vi "USRP Dummy (FPGA).vi"() -> ()   [LabVIEW 2016]
uses:
  <instrlib>/_niInstr/Register Bus/v1/FPGA/Public/Read Cmd Data.ctl
  <vilib>/Platform/TimedLoop/XDataNode/timing_clust.ctl
  <vilib>/Platform/TimedLoop/XDataNode/nitl_modes.ctl
  <vilib>/Platform/TimedLoop/XDataNode/wakeup.ctl
  <vilib>/rvi/Emulation/niFpgaSctlEmulationGetInTimedLoop.vi
  <vilib>/rvi/Emulation/niFpgaEmulationReportErrorSimple.vi
  <vilib>/rvi/Emulation/niFpgaGetClockAttributes.vi
  <vilib>/rvi/Emulation/niFpgaCriticalErrorInLSC.vi
  <vilib>/rvi/eio/common/nirviEmuTemplateMethod_errors.vi
  <vilib>/rvi/interface/RandomDataEmulation/niFpgaRandomDataHandleErrors.vi
  <vilib>/Platform/TimedLoop/XDataNode/XDataNode.xnode
  <vilib>/eio/EIONode/EIONode.xnode
  <vilib>/rvi/DataTransferAndStorage/Container/XNode/niFpgaContainer.xnode
  <vilib>/rvi/interface/RandomDataEmulation/nirviRandomDataFpgaReadWriteTemplate.vi
  <vilib>/Platform/TimedLoop/XDataNode/XDNodeRunTimeDep.lvlib
  <instrlib>/_niInstr/Register Bus/v1/FPGA/niInstr Register Bus v1 FPGA.lvlib
  <instrlib>/niUsrpRio/Config/v1/FPGA/niUsrpRio Config v1 FPGA.lvlib
  <instrlib>/_niInstr/Basic Elements/v1/FPGA/niInstr Basic Elements v1 FPGA.lvlib
panel:
  out "Min Space Available":u32
  out "Space Available":u32
  in  "Simulated Data Type":enum16{"Sequential", "Pseudo Random"}(ring)
  out "FPGA FIFO Depth":u32
  in  "Reset FPGA Transfer Count?":bool
  out "Send Status?":bool
  out "Samples Left to Write":u64
  in  "Number of Samples":u64
  in  "reg.host read.go rcvd 0":bool
  out "reg.notify host.go 0":bool
  in  "reg.notify host.go rcvd 0":bool
  out "reg.host read.data 0":T1
  in  "reg.reset 0":bool
  in  "RF 0/Rx/Enable":bool
  in  "RF 0/Tx/Enable":bool
  in  "RF 1/Rx/Enable":bool
  in  "RF 1/Tx/Enable":bool
  out "FPGA Transfer Count":u64
  in  "Send Data?":bool
  in  "Reset Total Timeouts?":bool
  out "Total Timeouts":u64
  out "Sticky Timeout?":bool
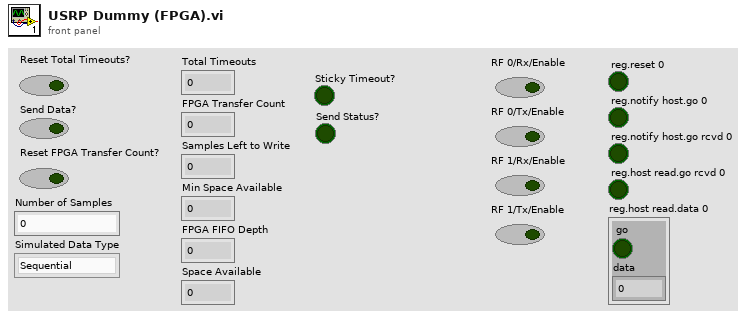
[diagram p1: front panel]
types:
  T1 = typedef "niInstr Register Bus v1 FPGA.lvlib/Read Cmd Data.ctl" = cluster{"go":bool, "data":u32}
  T2 = typedef "XDNodeRunTimeDep.lvlib/timing_clust.ctl" = cluster{"Expected End [f-1]":u64, "Actual End [f-1]":u64, "Finished Late? [f-1]":bool, "Expected End [i-1]":u64, "Actual End [i-1]":u64, "Finished Late? [i-1]":bool, "Expected Start [i]":u64, "Actual Start [i]":u64, "Expected Start [f]":u64, "Actual Start [f]":u64, "Source Name":string, "Structure Name":string, "Period":i64, "Deadline":i64, "Offset":i64, "Start":i64, "Priority":i32, "Timeout":i32, "Mode":T3, "Wakeup Reason":T4, "Error":errorcluster, "Source Type":string, "Secondary Source Type":string, "Global End Time":u64, "Global Start Time":u64, "Frame Duration":u64, "Iteration Duration":u64, "Assigned CPU":i32, "I/O Scan Engine Mode":u32}
  T3 = typedef "XDNodeRunTimeDep.lvlib/nitl_modes.ctl" = enum32{"No Change", "Process missed periods, maintain original phase", "Discard missed periods, maintain original phase", "Process missed periods, ignore original phase", "Discard missed periods, ignore original phase"}
  T4 = typedef "XDNodeRunTimeDep.lvlib/wakeup.ctl" = enum32{"Normal", "Aborted", "Asynchronous wakeup", "Timing source error", "Timed loop error", "Timeout"}
  T5 = cluster{"DAC FIFO Reset":refnum<k21>, "RF 0 Rx Swap IQ":refnum<k21>, "RF 0 Rx Negate I":refnum<k21>, "RF 0 Rx Negate Q":refnum<k21>, "RF 0 Rx Data Valid":refnum<k21>, "RF 0 Rx Data Ever Invalid":refnum<k21>, "clear RF 0 Rx Data Ever Invalid":refnum<k21>, "RF 0 Tx Swap IQ":refnum<k21>, "RF 0 Tx Negate I":refnum<k21>, "RF 0 Tx Negate Q":refnum<k21>, "RF 1 Rx Swap IQ":refnum<k21>, "RF 1 Rx Negate I":refnum<k21>, "RF 1 Rx Negate Q":refnum<k21>, "RF 1 Rx Data Valid":refnum<k21>, "RF 1 Rx Data Ever Invalid":refnum<k21>, "clear RF 1 Rx Data Ever Invalid":refnum<k21>, "RF 1 Tx Swap IQ":refnum<k21>, "RF 1 Tx Negate I":refnum<k21>, "RF 1 Tx Negate Q":refnum<k21>}
  T6 = typedef "niUsrpRio Synchronization v1 FPGA.lvlib/Resources.ctl" = cluster{"master":refnum<k21>, "meas.enable":refnum<k21>, "meas.ready":refnum<k21>, "meas.reset":refnum<k21>, "meas.arm":refnum<k21>, "meas.valid":refnum<k21>, "meas.value":refnum<k21>, "meas.oversample factor":refnum<k21>, "cptr":refnum<k21>, "cptr.adjust":refnum<k21>, "cptr.period":refnum<k21>}
  T7 = typedef "niUsrpRio Time v1 FPGA.lvlib/Time Resources.ctl" = cluster{"reset":refnum<k21>, "time":refnum<k21>, "time.previous cptr":refnum<k21>, "new time":refnum<k21>, "new time.when":refnum<k21>, "new time.set":refnum<k21>, "which edge of ref":refnum<k21>, "pps source":refnum<k21>, "internal pps period":refnum<k21>}
  T8 = typedef "niUsrpRio Time v1 FPGA.lvlib/Future Event Resources.ctl" = cluster{"reset":refnum<k21>, "future event.time":refnum<k21>, "future event.ready":refnum<k21>, "future event.set":refnum<k21>, "future event.clear":refnum<k21>, "future event.set in past":refnum<k21>}
  T9 = cluster{"time.resources":T7, "future event.resources":T8, "future event.resources":T8, "future event.resources":T8}
  T10 = typedef "niInstr Register Bus v1 FPGA.lvlib/Register Instruction.ctl" = cluster{"subsystem":u8, "address":u16, "data":u32, "valid":bool, "read":bool}
  T11 = typedef "niInstr Register Bus v1 FPGA.lvlib/Read Completion.ctl" = cluster{"data":u32, "valid":bool}
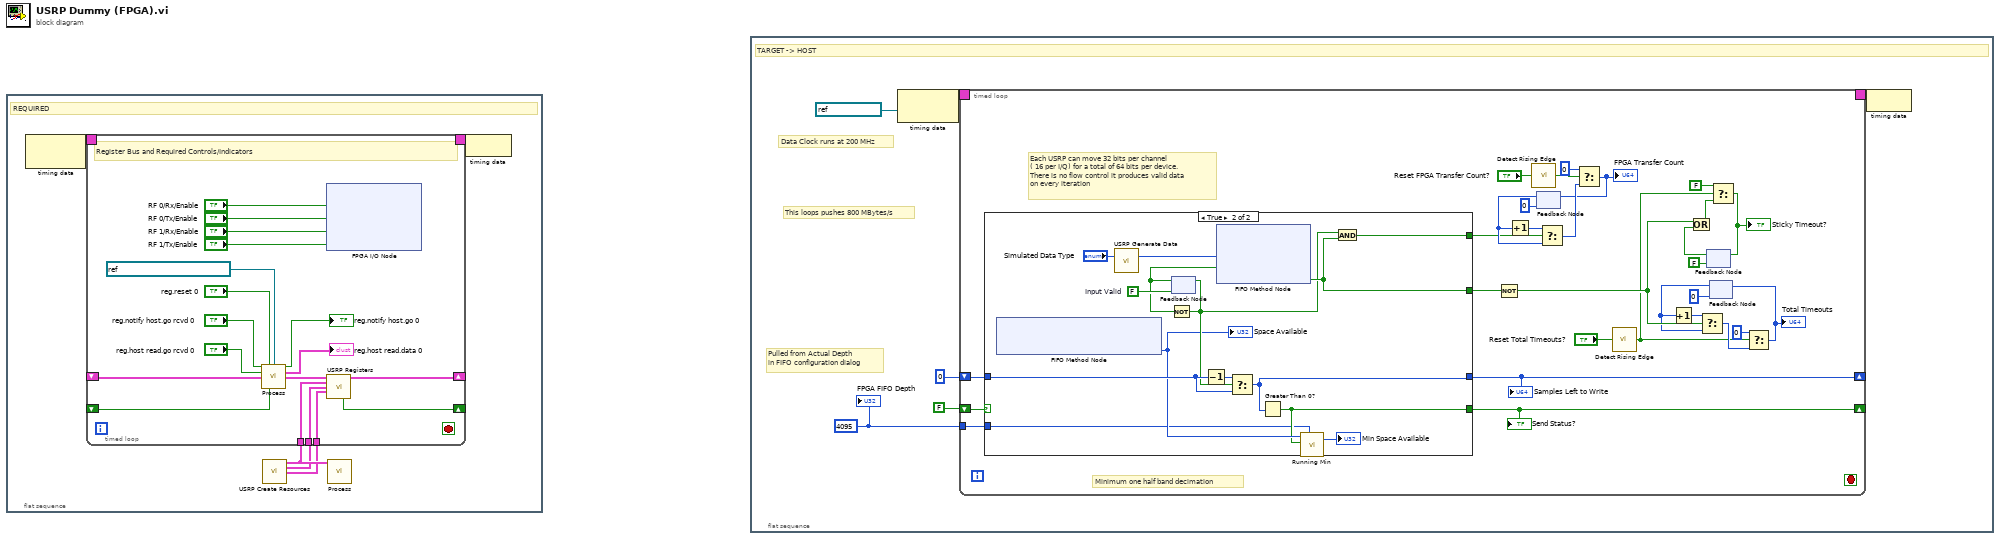
[diagram p0: block diagram]
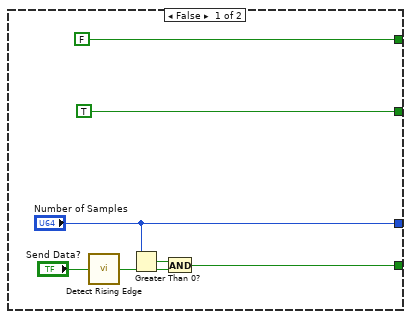
[diagram p2: hidden frame]
diagram:
  n1 = flat-sequence {
    frame #0 {
      # "REQUIRED"
      n2 = node-c288() -> (w5:T2)  [unwired: 1 in]
      n3 = call "USRP Create Resources.vi"() -> ("config.resources"=w3:T5, "sync.resources"=w2:T6, "time.resources"=w1:T9)  [unwired: 13 in]
      n4 = timed-loop "Register Bus and Required Controls/Indicators" {
        timing: w5 -> [_]
        timing-out: [_] -> w4
        shift-right: [w20] -> _
        shift-left: _ -> [w19]
        shift-right: [w14] -> _
        shift-left: _ -> [w18]
        tunnel: w3 -> [w12]
        tunnel: w2 -> [w11]
        tunnel: w1 -> [w10]
        stop <- _ stop-if-true
        # "Register Bus and Required Controls/Indicators"
        n5 = call <instrlib>:"Process.vi"("reg.notify host.go rcvd"="reg.notify host.go rcvd 0", "reg.reset"="reg.reset 0", "reg.host instruction fifo"=refnum<k21> "reg.host instruction fifo 0", "reg.host read.go rcvd"="reg.host read.go rcvd 0", "read completion"=w19, "ready for output"=w18) -> ("reg.notify host.go"=→"reg.notify host.go 0":bool, "reg.host read.data"=→"reg.host read.data 0":T1, "register instruction"=w13:T10)  [unwired: 7 in]
        n6 = xnode ("FPGA I/O Node")("RF 0/Rx/Enable"="RF 0/Rx/Enable", "RF 0/Tx/Enable"="RF 0/Tx/Enable", "RF 1/Rx/Enable"="RF 1/Rx/Enable", "RF 1/Tx/Enable"="RF 1/Tx/Enable") -> ()  [unwired: 4 in, 4 out]
        n7 = call "USRP Registers.vi"("register instruction"=w13, "config.resources"=w12, "sync.resources"=w11, "time.resources"=w10) -> ("read completion out"=w20:T11, "ready for input"=w14:bool)  [unwired: 10 in]
      }
      n8 = call <instrlib>:"Process.vi"("resources"=w3) -> ()  [unwired: 15 in]
      n9 = node-c288(w4) -> ()
    }
  }
  n10 = flat-sequence {
    frame #0 {
      w28 = u32 4095 ("FPGA FIFO Depth")
      # "Pulled from Actual Depth\nin FIFO configuration dialog"
      # "This loops pushes 800 MBytes/s"
      # "Data Clock runs at 200 MHz"
      # "TARGET -> HOST"
      n11 = node-c288(refnum<k21> "Data Clock" ("Source Name")) -> (w33:T2)
      n12 = timed-loop {
        timing: w33 -> [_]
        timing-out: [_] -> w32
        shift-right: [w50] -> _
        shift-left: FALSE ("send data?") -> [w49]
        shift-right: [w47] -> _
        shift-left: u64 0 ("samples to write") -> [w48]
        tunnel: w28 -> [w38]
        stop <- _ stop-if-true
        # "Each USRP can move 32 bits per channel\n( 16 per I/Q) for a total of 64 bits per device.\nThere is no flow control it produces valid data\non every iteration"
        # "Minimum one half band decimation"
        n13 = case shown="True" w49 {
          tunnel: [FALSE ("Timed Out?") w75] -> w53
          tunnel: [TRUE ("Timed Out?") w83] -> w52
          tunnel: [w65 w72] -> w50
          tunnel: w48 -> [_ w78]
          tunnel: ["Number of Samples" w79] -> w47
          tunnel: w38 -> [_ w71]
          frame False {
            n14 = call <instrlib>:"Detect Rising Edge.vi"("signal"="Send Data?") -> ("edge detected"=w66:bool)  [unwired: 14 in]
            n15 = Greater Than 0?(x="Number of Samples") -> (x > 0?=w64:bool)
            n16 = And(x=w64, y=w66) -> (x .and. y?=w65:bool)
          }
          frame True {
            w82 = FALSE  # Input Valid
            n17 = xnode ("FIFO Method Node")() -> ("Number of Elements to Write"=w73:u32)  [unwired: 1 in, 1 out]
            "Space Available" <- w73
            n18 = call "USRP Generate Data.vi"("Enum"="Simulated Data Type") -> ("Data"=w77:u64)  [unwired: 14 in]
            n19 = feedback #1(w82) -> (w81:bool)
            n20 = Not(x=w81) -> (.not. x?=w74:bool)
            n21 = feedback-in #1(w74) -> ()
            n22 = Decrement(x=w78) -> (x-1=w80:u64)
            n23 = xnode ("FIFO Method Node")("Element"=w77, "Input Valid"=w81) -> ("Ready for Input"=w83:bool)  [unwired: 1 in, 1 out]
            n24 = Select(t=w80, s=w74, f=w78) -> (s? t:f=w79:u64)
            n25 = Greater Than 0?(x=w79) -> (x > 0?=w72:bool)
            n26 = call "Running Min.vi"("Starting Min"=w71, "Reset"=w72, "Next Value"=w73) -> ("Running Min"=→"Min Space Available":u32)  [unwired: 4 in]
            n27 = And(x=w74, y=w83) -> (x .and. y?=w75:bool)
          }
        }
        "Samples Left to Write" <- w47
        "Send Status?" <- w50
        n28 = Not(x=w52) -> (.not. x?=w51:bool)
        n29 = call <instrlib>:"Detect Rising Edge.vi"("signal"="Reset FPGA Transfer Count?") -> ("edge detected"=w39:bool)  [unwired: 14 in]
        n30 = feedback #2(u64 0) -> (w55:u64)
        n31 = Increment(x=w55) -> (x+1=w54:u64)
        n32 = Select(t=w54, s=w53, f=w55) -> (s? t:f=w42:u64)
        n33 = Select(t=u64 0, s=w39, f=w42) -> (s? t:f=w41:u64)
        "FPGA Transfer Count" <- w41
        n34 = feedback-in #2(w41) -> ()
        n35 = call <instrlib>:"Detect Rising Edge.vi"("signal"="Reset Total Timeouts?") -> ("edge detected"=w37:bool)  [unwired: 14 in]
        n36 = feedback #3(FALSE) -> (w58:bool)
        n37 = Or(x=w51, y=w58) -> (x .or. y?=w36:bool)
        n38 = feedback #4(u64 0) -> (w46:u64)
        n39 = Increment(x=w46) -> (x+1=w45:u64)
        n40 = Select(t=w45, s=w51, f=w46) -> (s? t:f=w61:u64)
        n41 = Select(t=FALSE, s=w37, f=w36) -> (s? t:f=w35:bool)
        "Sticky Timeout?" <- w35
        n42 = feedback-in #3(w35) -> ()
        n43 = Select(t=u64 0, s=w37, f=w61) -> (s? t:f=w60:u64)
        "Total Timeouts" <- w60
        n44 = feedback-in #4(w60) -> ()
      }
      n45 = node-c288(w32) -> ()
      "FPGA FIFO Depth" <- w28
    }
  }
